vi "Gpad Target Select.vi"(9 "Left Hoop":bool, 10 "Right Hoop":bool, 11 "Top Hoop":bool) -> (3 "Hoop Select":T1(ring))   [LabVIEW 2011]
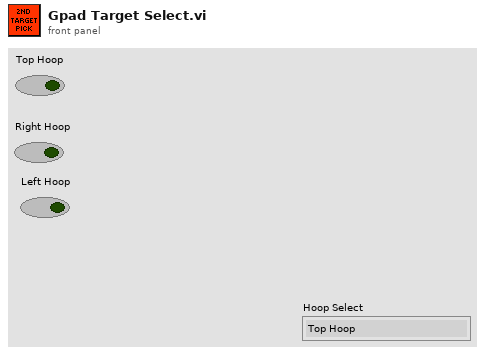
[diagram p1: front panel]
types:
  T1 = enum32{"Top Hoop", "Bottom Hoop", "Left Hoop", "Right Hoop"}
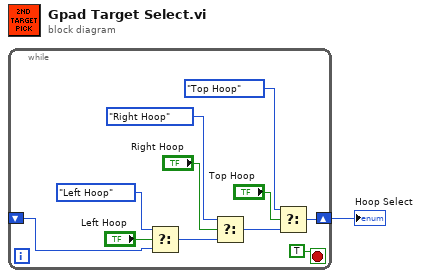
[diagram p0: block diagram]
diagram:
  n1 = while {
    shift-right: [w4] -> w1
    shift-left: _ -> [w2]
    stop <- TRUE stop-if-true
    n2 = Select(t=T1."Left Hoop" ("Radio Buttons"), s="Left Hoop", f=w2) -> (s? t:f=w9:T1)
    n3 = Select(t=T1."Right Hoop" ("Radio Buttons"), s="Right Hoop", f=w9) -> (s? t:f=w8:T1)
    n4 = Select(t=T1."Top Hoop" ("Radio Buttons"), s="Top Hoop", f=w8) -> (s? t:f=w4:T1)
  }
  "Hoop Select" <- w1
